vi "Estatus Servicio.vi"(11 "Lista servicios":string[](array[string])) -> (3 "Servicios Estatus":string[][](array[string]))   [LabVIEW 2020, in "Manejador Turnos.lvlib"]
uses:
  Manejador Turnos.lvlib
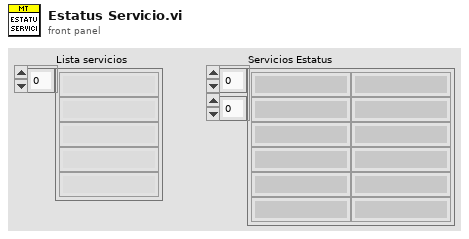
[diagram p1: front panel]
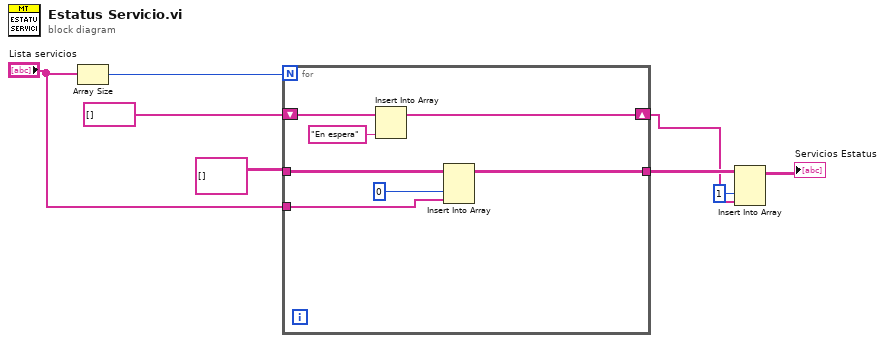
[diagram p0: block diagram]
diagram:
  n1 = Array Size(array="Lista servicios") -> (size(s)=w8:i32)
  n2 = for {
    N: w8 -> [_]
    shift-right: [w13] -> w3
    shift-left: string[] [] ("array") -> [w15]
    tunnel: string[][] [] -> [w12]
    tunnel: "Lista servicios" -> [w10]
    tunnel: [w9] -> w4
    n3 = Insert Into Array(array=w15, new element="En espera" ("new element/subarray")) -> (w13:string[])  [unwired: 1 in]
    n4 = Insert Into Array(array=w12, index (col)=0 ("disabled index (col)"), new element=w10) -> (w9:string[][])  [unwired: 1 in]
  }
  n5 = Insert Into Array(array=w4, index (col)=1 ("disabled index (col)"), new element=w3) -> (→"Servicios Estatus":string[][])  [unwired: 1 in]
